vi "Format RunningInstancesItemType_LVXML.vi"(8 "error in (no error)":errorcluster, 10 "valueXmlData":T2, 11 "AWS_EC2 in":refnum<class "AWS_EC2.lvclass">) -> (0 "error out":errorcluster, 2 "Array":T3[](array[typedef]), 3 "AWS_EC2 out":refnum<class "AWS_EC2.lvclass">)   [LabVIEW 2014, in "AWS_EC2.lvlib" / "AWS_EC2.lvclass"]
uses:
  AWS_EC2.lvclass
  EC2 Datatypes/RunningInstancesItemsType.ctl
  EC2 Datatypes/InstanceStateType.ctl
  EC2 Datatypes/ProductCodeSetItemType.ctl
  EC2 Datatypes/PlacementResponseType.ctl
  EC2 Datatypes/GroupItemTypeSet.ctl
  EC2 Datatypes/GroupItemType.ctl
  EC2 Datatypes/StateReasonType.ctl
  EC2 Datatypes/InstanceBlockDeviceMappingResponseItemType.ctl
  EC2 Datatypes/EbsInstanceBlockDeviceMappingResponseType.ctl
  EC2 Datatypes/ResourceTagSetItemType.ctl
  EC2 Datatypes/InstanceNetworkInterfaceSetItemType.ctl
  EC2 Datatypes/InstanceNetworkInterfaceAttachmentType.ctl
  EC2 Datatypes/InstanceNetworkInterfaceAssociationType.ctl
  EC2 Datatypes/InstancePrivateIpAddressesSetItemType.ctl
  EC2 Datatypes/IamInstanceProfileResponseType.ctl
  lv-xml-parser/r0/trunk/VI Source/EventType.ctl
  lv-xml-parser/r0/trunk/VI Source/LV XML Parser.lvlib
  AWS_EC2.lvlib
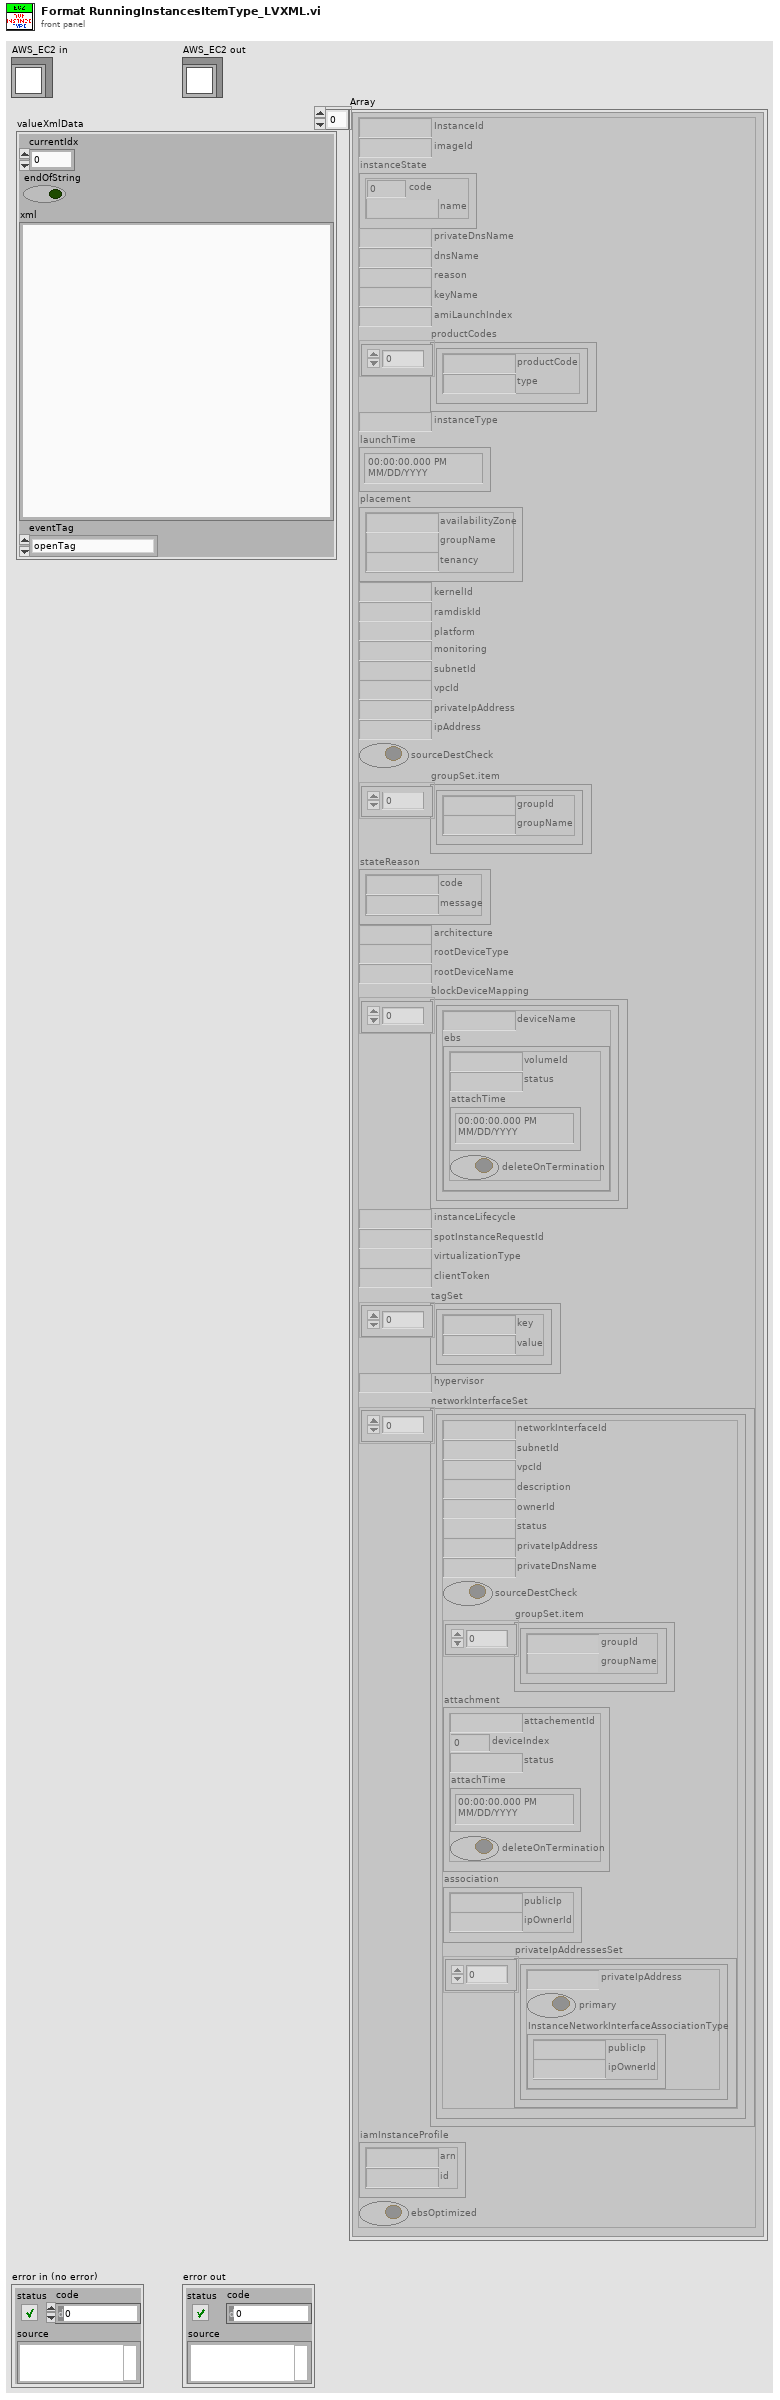
[diagram p1: front panel]
types:
  T1 = typedef "LV XML Parser.lvlib/EventType.ctl" = enum16{"openTag", "endOpenTag", "closeTag", "comment", "endComment", "endOfFile", "attribute", "startXml"}
  T2 = cluster{"currentIdx":i32, "endOfString":bool, "xml":string, "eventTag":T1}
  T3 = typedef "AWS_EC2.lvlib/RunningInstancesItemsType.ctl" = cluster{"InstanceId":string, "imageId":string, "instanceState":T4, "privateDnsName":string, "dnsName":string, "reason":string, "keyName":string, "amiLaunchIndex":string, "productCodes":T5[], "instanceType":string, "launchTime":timestamp, "placement":T6, "kernelId":string, "ramdiskId":string, "platform":string, "monitoring":string, "subnetId":string, "vpcId":string, "privateIpAddress":string, "ipAddress":string, "sourceDestCheck":bool, "groupSet.item":T7, "stateReason":T9, "architecture":string, "rootDeviceType":string, "rootDeviceName":string, "blockDeviceMapping":T10[], "instanceLifecycle":string, "spotInstanceRequestId":string, "virtualizationType":string, "clientToken":string, "tagSet":T12[], "hypervisor":string, "networkInterfaceSet":T13[], "iamInstanceProfile":T17, "ebsOptimized":bool}
  T4 = typedef "AWS_EC2.lvlib/InstanceStateType.ctl" = cluster{"code":i16, "name":string}
  T5 = typedef "AWS_EC2.lvlib/ProductCodeSetItemType.ctl" = cluster{"productCode":string, "type":string}
  T6 = typedef "AWS_EC2.lvlib/PlacementResponseType.ctl" = cluster{"availabilityZone":string, "groupName":string, "tenancy":string}
  T7 = typedef "AWS_EC2.lvlib/GroupItemTypeSet.ctl" = T8[]
  T8 = typedef "AWS_EC2.lvlib/GroupItemType.ctl" = cluster{"groupId":string, "groupName":string}
  T9 = typedef "AWS_EC2.lvlib/StateReasonType.ctl" = cluster{"code":string, "message":string}
  T10 = typedef "AWS_EC2.lvlib/InstanceBlockDeviceMappingResponseItemType.ctl" = cluster{"deviceName":string, "ebs":T11}
  T11 = typedef "AWS_EC2.lvlib/EbsInstanceBlockDeviceMappingResponseType.ctl" = cluster{"volumeId":string, "status":string, "attachTime":timestamp, "deleteOnTermination":bool}
  T12 = typedef "AWS_EC2.lvlib/ResourceTagSetItemType.ctl" = cluster{"key":string, "value":string}
  T13 = typedef "AWS_EC2.lvlib/InstanceNetworkInterfaceSetItemType.ctl" = cluster{"networkInterfaceId":string, "subnetId":string, "vpcId":string, "description":string, "ownerId":string, "status":string, "privateIpAddress":string, "privateDnsName":string, "sourceDestCheck":bool, "groupSet.item":T7, "attachment":T14, "association":T15, "privateIpAddressesSet":T16[]}
  T14 = typedef "AWS_EC2.lvlib/InstanceNetworkInterfaceAttachmentType.ctl" = cluster{"attachementId":string, "deviceIndex":i32, "status":string, "attachTime":timestamp, "deleteOnTermination":bool}
  T15 = typedef "AWS_EC2.lvlib/InstanceNetworkInterfaceAssociationType.ctl" = cluster{"publicIp":string, "ipOwnerId":string}
  T16 = typedef "AWS_EC2.lvlib/InstancePrivateIpAddressesSetItemType.ctl" = cluster{"privateIpAddress":string, "primary":bool, "InstanceNetworkInterfaceAssociationType":T15}
  T17 = typedef "AWS_EC2.lvlib/IamInstanceProfileResponseType.ctl" = cluster{"arn":string, "id":string}
  T18 = cluster{"namespaceUri":string, "localName":string}
  T19 = cluster{"Attributes":cluster{"localName":string, "namespaceUri":string, "value":string}[], "localName":string, "namespaceUri":string, "valueXmlData":cluster{"currentIdx":i64, "endOfString":bool, "xml":string, "eventTag":T1}}[]
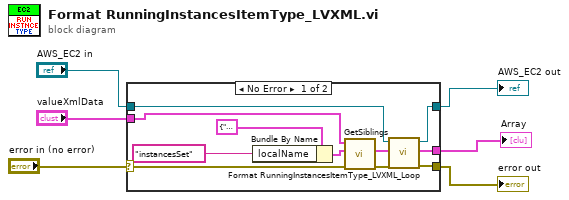
[diagram p0: block diagram]
diagram:
  n1 = case shown="No Error" "error in (no error)" {
    selector: "error in (no error)" -> [w13 w18]
    tunnel: [w9 w19] -> w4
    tunnel: "AWS_EC2 in" -> [w10 w19]
    tunnel: [w7 w18] -> w2
    tunnel: "valueXmlData" -> [w17 _]
    tunnel: [w8 _] -> w6
    frame No Error {
      n2 = Bundle By Name(cluster=T18 {"namespaceUri"="", "localName"=""} ("limitToTag"), "localName"="instancesSet" ("Tag name")) -> (w14:T18)
      n3 = call "GetSiblings.vi"("error in (no error)"=w13, "limitToTag"=w14, "xmlData"=w17) -> ("error out"=w12:errorcluster, "Siblings"=w11:T19)  [unwired: 7 in]
      n4 = call "Format RunningInstancesItemType_LVXML_Loop.vi"("error in (no error)"=w12, "Siblings in"=w11, "AWS_EC2 in"=w10) -> ("error out"=w7:errorcluster, "Array"=w8:T3[], "AWS_EC2 out"=w9:refnum<class "AWS_EC2.lvclass">)  [unwired: 6 in]
    }
    frame Error {
    }
  }
  "Array" <- w6
  "AWS_EC2 out" <- w4
  "error out" <- w2
